vi "FA_SharedVariablesFilePath.vi"() -> (3 "appended path":path)   [LabVIEW 2014, in "FA_SharedVariables.lvlib"]
doc: "Builds the path to the shared variable XML file (Information.xml)"
uses:
  FA_SharedVariables.lvlib
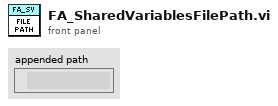
[diagram p1: front panel]
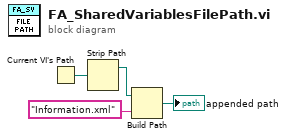
[diagram p0: block diagram]
diagram:
  n1 = Current VI's Path() -> (path=w2:path)
  n2 = Strip Path(path=w2) -> (stripped path=w3:path)  [unwired: 1 out]
  n3 = Build Path(base path=w3, name or relative path="Information.xml" ("XML File Name")) -> (appended path=→"appended path":path)
